vi "init.vi"(8 "error in":errorcluster, 10 "TBM module configuration in":refnum<class "TBM module configuration.lvclass">, 11 "dds runtime in":refnum<class "dds runtime.lvclass">) -> (0 "error out":errorcluster, 1 "data allocations":T1, 2 "execution settings":T4, 3 "dds runtime out":refnum<class "dds runtime.lvclass">)   [LabVIEW 2013, in "dds runtime.lvclass"]
doc: "Provides an interface for initializing a module at runtime. While this interface performs no operations, a child should provide an override which may open any necessary references or sessions, allocate necessary memory, and perform any final configuration validataion before providing the full configuration <b>execution data</b> to the calling process."
uses:
  dds runtime.lvclass
  <vilib>/NI/Tag Bus Module Framework/module configuration/TBM module configuration.lvclass
  <vilib>/NI/Tag Bus Module Framework/runtime/execution settings.ctl
  <vilib>/NI/Tag Bus Module Framework/channel/data tables.ctl
  <vilib>/NI/Tag Bus/dictionary/data dictionary.lvclass
  <vilib>/NI/Tag Bus/dictionary table pair.ctl
  <vilib>/NI/Tag Bus/table/data table.ctl
  configuration/dds configuration.lvclass
  configuration/dds configuration.lvclass/dds configuration.ctl
  <vilib>/NI/Tag Bus Module Framework/channel/TBM channel.lvclass/TBM channel.ctl
  dds runtime.lvclass/dds runtime.ctl
  <vilib>/NI/Tag Bus/tag/Data Type.ctl
  <vilib>/NI/Tag Bus/tag/tag descriptor.lvclass/tag descriptor.ctl
  <vilib>/RTI DDS Toolkit for LabVIEW/VIs/AdvancedCreateReader_NumDbl.vi
  <vilib>/RTI DDS Toolkit for LabVIEW/VIs/AdvancedCreateReader_NumSgl.vi
  <vilib>/RTI DDS Toolkit for LabVIEW/VIs/AdvancedCreateReader_NumI64.vi
  <vilib>/RTI DDS Toolkit for LabVIEW/VIs/AdvancedCreateReader_NumI32.vi
  <vilib>/RTI DDS Toolkit for LabVIEW/VIs/AdvancedCreateReader_NumI16.vi
  <vilib>/RTI DDS Toolkit for LabVIEW/VIs/AdvancedCreateReader_NumI8.vi
  <vilib>/RTI DDS Toolkit for LabVIEW/VIs/AdvancedCreateReader_NumU64.vi
  <vilib>/RTI DDS Toolkit for LabVIEW/VIs/AdvancedCreateReader_NumU32.vi
  <vilib>/RTI DDS Toolkit for LabVIEW/VIs/AdvancedCreateReader_NumU16.vi
  <vilib>/RTI DDS Toolkit for LabVIEW/VIs/AdvancedCreateReader_NumU8.vi
  <vilib>/RTI DDS Toolkit for LabVIEW/VIs/AdvancedCreateReader_Bool.vi
  <vilib>/RTI DDS Toolkit for LabVIEW/VIs/AdvancedCreateReader_String.vi
  <vilib>/RTI DDS Toolkit for LabVIEW/VIs/AdvancedCreateWriter_NumDbl.vi
  <vilib>/RTI DDS Toolkit for LabVIEW/VIs/AdvancedCreateWriter_NumSgl.vi
  <vilib>/RTI DDS Toolkit for LabVIEW/VIs/AdvancedCreateWriter_NumI64.vi
  <vilib>/RTI DDS Toolkit for LabVIEW/VIs/AdvancedCreateWriter_NumI32.vi
  <vilib>/RTI DDS Toolkit for LabVIEW/VIs/AdvancedCreateWriter_NumI16.vi
  <vilib>/RTI DDS Toolkit for LabVIEW/VIs/AdvancedCreateWriter_NumI8.vi
  <vilib>/RTI DDS Toolkit for LabVIEW/VIs/AdvancedCreateWriter_NumU64.vi
  <vilib>/RTI DDS Toolkit for LabVIEW/VIs/AdvancedCreateWriter_NumU32.vi
  <vilib>/RTI DDS Toolkit for LabVIEW/VIs/AdvancedCreateWriter_NumU16.vi
  <vilib>/RTI DDS Toolkit for LabVIEW/VIs/AdvancedCreateWriter_NumU8.vi
  <vilib>/RTI DDS Toolkit for LabVIEW/VIs/AdvancedCreateWriter_Bool.vi
  <vilib>/RTI DDS Toolkit for LabVIEW/VIs/AdvancedCreateWriter_String.vi
  <vilib>/NI/Tag Bus Module Framework/channel/TBM channel.lvclass
  <vilib>/NI/Tag Bus Module Framework/runtime/TBM module execution interface.lvclass
  <vilib>/NI/Tag Bus/tag/tag descriptor.lvclass
  <vilib>/RTI DDS Toolkit for LabVIEW/Library/LVDDS_library.lvlib
  <vilib>/NI/Tag Bus/tag bus.lvlib
  <vilib>/NI/Tag Bus/table/data table.lvlib
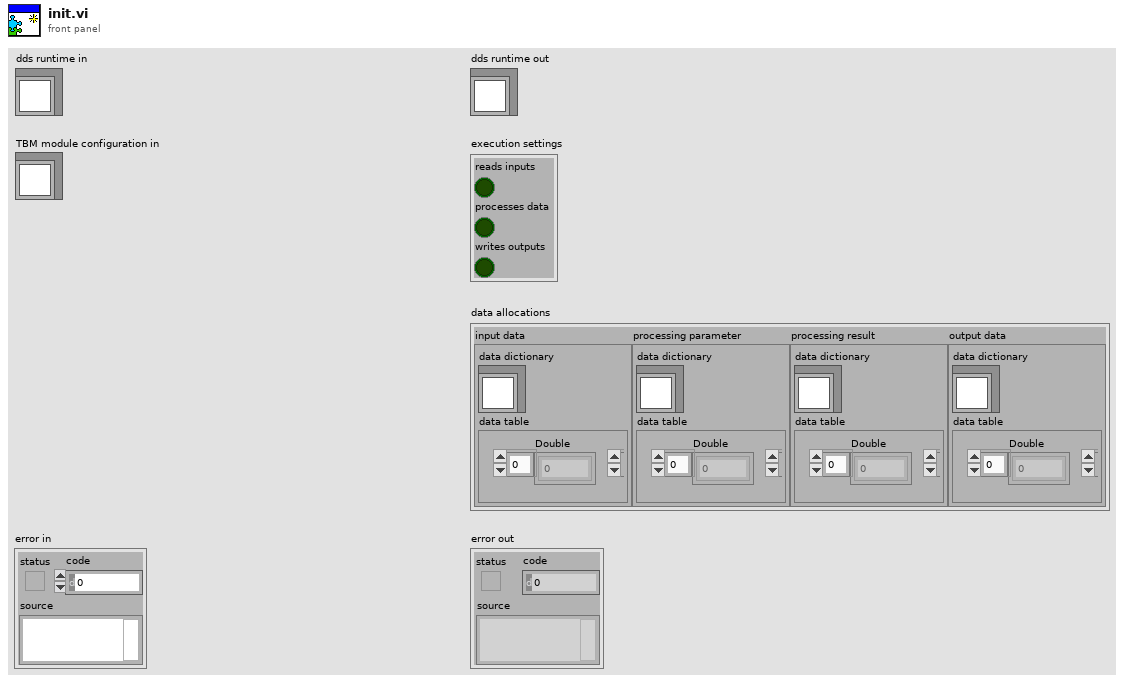
[diagram p1: front panel]
types:
  T1 = typedef "TBM channel.lvclass/data tables.ctl" = cluster{"input data":T2, "processing parameter":T2, "processing result":T2, "output data":T2}
  T2 = typedef "tag bus.lvlib/dictionary table pair.ctl" = cluster{"data dictionary":refnum<class "data dictionary.lvclass">, "data table":T3}
  T3 = typedef "tag bus.lvlib/data table.lvlib/data table.ctl" = cluster{"Double":dbl[], "Single":sgl[], "I64":i64[], "I32":i32[], "I16":i16[], "I8":i8[], "U64":u64[], "U32":u32[], "U16":u16[], "U8":u8[], "Boolean":bool[], "String":string[], "Array of Double":cluster{"DBL Array":dbl[]}[], "Array of Single":cluster{"SGL Array":sgl[]}[], "Array of I64":cluster{"I64 Array":i64[]}[], "Array of I32":cluster{"I32 Array":i32[]}[], "Array of I16":cluster{"I16 Array":i16[]}[], "Array of I8":cluster{"I8 Array":i8[]}[], "Array of U64":cluster{"U64 Array":u64[]}[], "Array of U32":cluster{"U32 Array":u32[]}[], "Array of U16":cluster{"U16 Array":u16[]}[], "Array of U8":cluster{"U8 Array":u8[]}[], "Array of Boolean":cluster{"Boolean Array":bool[]}[], "Array of String":cluster{"String Array":string[]}[]}
  T4 = typedef "TBM module execution interface.lvclass/execution settings.ctl" = cluster{"reads inputs":bool, "processes data":bool, "writes outputs":bool}
  T5 = typedef "tag bus.lvlib/tag descriptor.lvclass/Data Type.ctl" = enum16{"Double", "Single", "I64", "I32", "I16", "I8", "U64", "U32", "U16", "U8", "Boolean", "String", "Array of Double", "Array of Single", "Array of I64", "Array of I32", "Array of I16", "Array of I8", "Array of U64", "Array of U32", "Array of U16", "Array of U8", "Array of Boolean", "Array of String"}
  T6 = cluster{"index":i32, "data type":T5, "ref num":u64, "new samples only":bool, "query condition":string}
  T7 = cluster{"index":i32, "data type":T5, "ref num":u64}
  T8 = typedef "dds configuration.lvclass/Line.ctl" = cluster{"channel":refnum<class "TBM channel.lvclass">, "DDS topic":string, "DDS Domain":u32, "advanced configuration":T9}
  T9 = typedef "LVDDS_library.lvlib/RTI DDS Advanced Reader Configuration.ctl" = cluster{"typeName":string, "keyName":string, "domainParticipantQoSProfile":string, "dataReaderQoSProfile":string, "forceNewDomainParticipant?":bool, "forceArrayMapping?":bool, "forceExclusiveReader?":bool, "forceRead? (only ExclusiveReader)":bool, "forceUnboundedString?":bool}
  T10 = typedef "TBM channel.lvclass/channel classification.ctl" = enum16{"input data", "output data", "processing parameter", "processing result"}
  T11 = cluster{"index":i32, "data type":T5, "ref num":u64, "new samples only":bool, "query condition":string}[]
  T12 = cluster{"index":i32, "data type":T5, "ref num":u64}[]
  T13 = typedef "LVDDS_library.lvlib/RTI DDS Advanced Writer Configuration.ctl" = cluster{"typeName":string, "keyName":string, "domainParticipantQoSProfile":string, "dataWriterQoSProfile":string, "forceNewDomainParticipant?":bool, "forceArrayMapping?":bool, "forceUnboundedString?":bool}
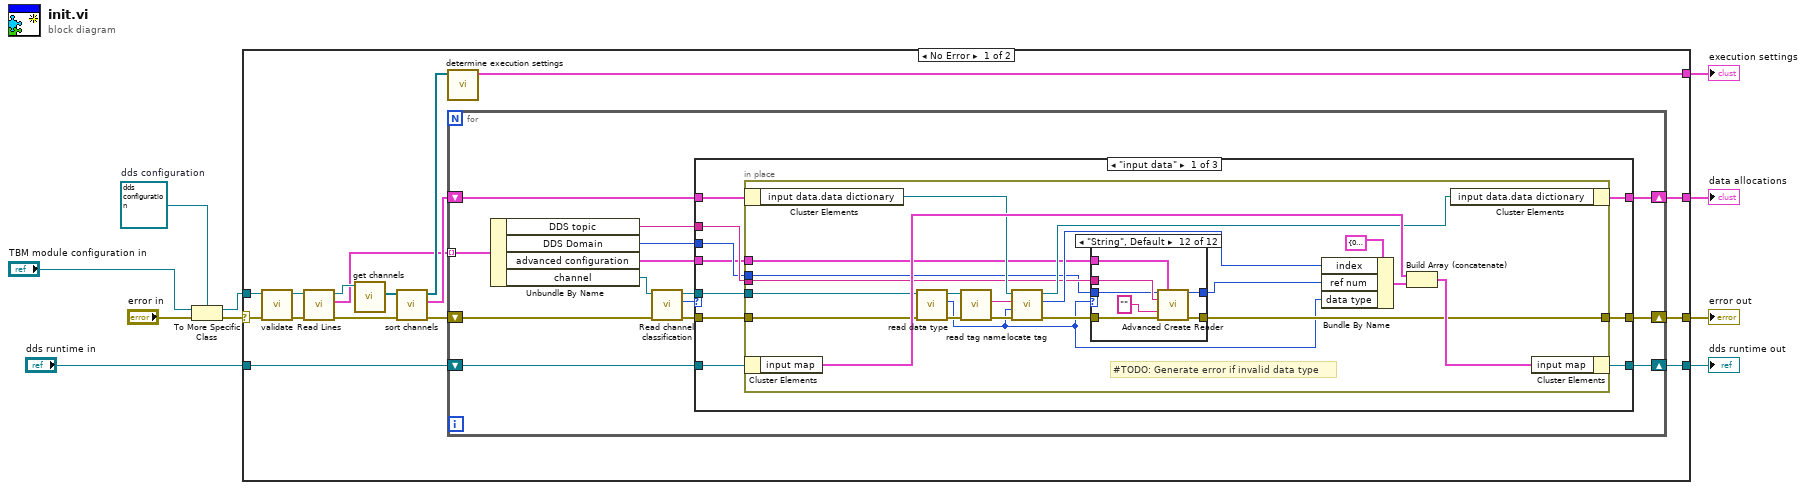
[diagram p0: block diagram]
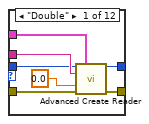
[diagram p2: hidden frame]
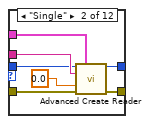
[diagram p3: hidden frame]
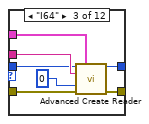
[diagram p4: hidden frame]
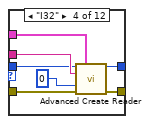
[diagram p5: hidden frame]
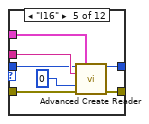
[diagram p6: hidden frame]
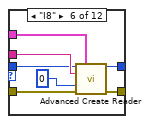
[diagram p7: hidden frame]
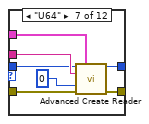
[diagram p8: hidden frame]
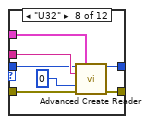
[diagram p9: hidden frame]
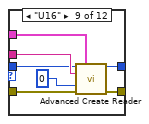
[diagram p10: hidden frame]
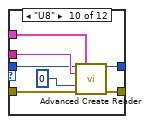
[diagram p11: hidden frame]
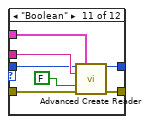
[diagram p12: hidden frame]
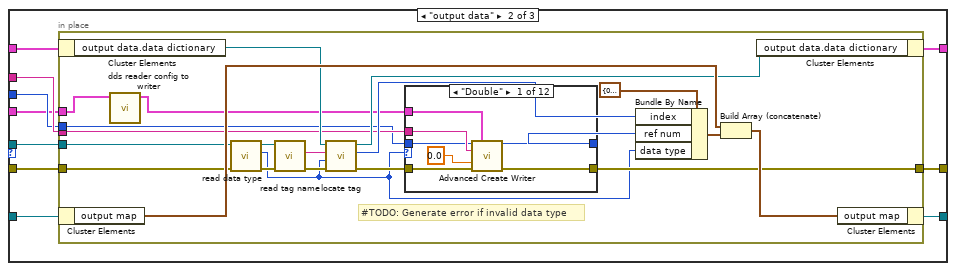
[diagram p13: hidden frame]
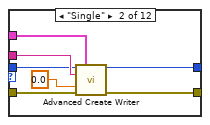
[diagram p14: hidden frame]
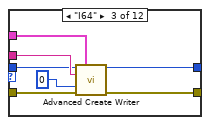
[diagram p15: hidden frame]
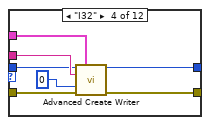
[diagram p16: hidden frame]
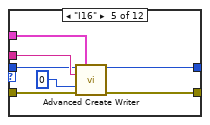
[diagram p17: hidden frame]
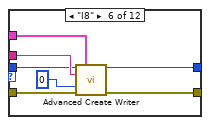
[diagram p18: hidden frame]
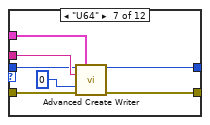
[diagram p19: hidden frame]
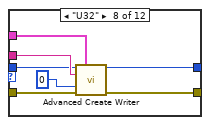
[diagram p20: hidden frame]
diagram:
  w8 = refnum<class "dds configuration.lvclass"> refnum  # dds configuration
  n1 = To More Specific Class(target class=w8, reference="TBM module configuration in", error in="error in") -> (specific class reference=w9:refnum<class "dds configuration.lvclass">, error out=w10:errorcluster)
  n2 = case shown="No Error" w10 {
    selector: w10 -> [w25 w273]
    tunnel: w9 -> [w24 _]
    tunnel: "dds runtime in" -> [w23 w274]
    tunnel: [w22 w274] -> w4
    tunnel: [w12 w273] -> w3
    tunnel: [w11 _] -> w1
    tunnel: [w26 _] -> w2
    frame No Error {
      n3 = call-dynamic "validate.vi"("error in"=w25, "dds configuration in"=w24) -> ("error out"=w17:errorcluster, "dds configuration out"=w18:refnum<class "dds configuration.lvclass">)  [unwired: 8 in]
      n4 = call "Read Lines.vi"("error in (no error)"=w17, "dds configuration in"=w18) -> ("error out"=w16:errorcluster, "Lines"=w14:T8[], "dds configuration out"=w15:refnum<class "dds configuration.lvclass">)  [unwired: 7 in]
      n5 = call-dynamic "get channels.vi"("dds configuration in"=w15) -> ("channels"=w21:refnum<class "TBM channel.lvclass">[])  [unwired: 9 in, 1 out]
      n6 = call <vilib>:"sort channels.vi"("error in"=w16, "channels in"=w21) -> ("error out"=w13:errorcluster, "data allocations"=w19:T1, "channels out"=w20:refnum<class "TBM channel.lvclass">[])  [unwired: 7 in]
      n7 = call <vilib>:"determine execution settings.vi"("channels"=w20) -> ("execution settings"=w26:T4)  [unwired: 10 in]
      n8 = for {
        shift-right: [w37] -> w22
        shift-left: w23 -> [w40]
        tunnel: w14 -> [w34] mode=indexing
        shift-right: [w29] -> w12
        shift-left: w13 -> [w30]
        shift-right: [w27] -> w11
        shift-left: w19 -> [w35]
        n9 = Unbundle By Name(w34) -> ("DDS topic"=w33:string, "DDS Domain"=w32:u32, "advanced configuration"=w31:T9, "channel"=w28:refnum<class "TBM channel.lvclass">)
        n10 = call <vilib>:"Read channel classification.vi"("error in"=w30, "channel in"=w28) -> ("error out"=w36:errorcluster, "channel classification"=w39:T10, "channel out"=w38:refnum<class "TBM channel.lvclass">)  [unwired: 7 in]
        n11 = case shown="\"input data\"" w39 {
          tunnel: w40 -> [w50 w164 w270]
          tunnel: w38 -> [w47 w161 _]
          tunnel: [w49 w163 w270] -> w37
          tunnel: w36 -> [w48 w162 w271]
          tunnel: w35 -> [w46 w160 w272]
          tunnel: w33 -> [w45 w159 _]
          tunnel: w32 -> [w44 w158 _]
          tunnel: w31 -> [w43 w157 _]
          tunnel: [w42 w156 w271] -> w29
          tunnel: [w41 w155 w272] -> w27
          frame "input data" {
            n12 = in-place {
              in-place-border: w48 -> [w68]
              in-place-border: w47 -> [w66]
              in-place-border: w45 -> [w58]
              in-place-border: w44 -> [w57]
              in-place-border: w43 -> [w56]
              in-place-border: [w54] -> w42
              # "#TODO: Generate error if invalid data type"
              n13 = in-place-cluster #1(w46) -> ("input data.data dictionary"=w65:refnum<class "data dictionary.lvclass">)
              n14 = in-place-cluster #2(w50) -> ("input map"=w70:T11)
              n15 = call <vilib>:"read data type.vi"("error in"=w68, "system tag in"=w66) -> ("error out"=w62:errorcluster, "data type"=w52:T5, "system tag out"=w63:refnum<class "TBM channel.lvclass">)  [unwired: 7 in]
              n16 = call <vilib>:"read tag name.vi"("error in"=w62, "system tag in"=w63) -> ("error out"=w55:errorcluster, "name"=w61:string)  [unwired: 7 in, 1 out]
              n17 = call <vilib>:"locate tag.vi"("error in"=w55, "data type"=w52, "name"=w61, "data dictionary in"=w65) -> ("error out"=w60:errorcluster, "index"=w59:i32, "data dictionary out"=w64:refnum<class "data dictionary.lvclass">)  [unwired: 5 in]
              n18 = case shown="\"String\", Default" w52 {
                tunnel: [w77 w84 w91 w98 w105 w112 w119 w126 w133 w140 w147 w154] -> w53
                tunnel: w60 -> [w75 w82 w89 w96 w103 w110 w117 w124 w131 w138 w145 w152]
                tunnel: [w74 w81 w88 w95 w102 w109 w116 w123 w130 w137 w144 w151] -> w54
                tunnel: w58 -> [w73 w80 w87 w94 w101 w108 w115 w122 w129 w136 w143 w150]
                tunnel: w57 -> [w72 w79 w86 w93 w100 w107 w114 w121 w128 w135 w142 w149]
                tunnel: w56 -> [w71 w78 w85 w92 w99 w106 w113 w120 w127 w134 w141 w148]
                frame "Double" {
                  n19 = call-poly <vilib>:"Advanced Create Reader.vi"("domain id"=w72, "advanced reader configuration"=w71, "topic name"=w73, "data type"=0.0, "error in (no error)"=w75) -> ("ref num"=w77:u64, "error out"=w74:errorcluster)  [unwired: 9 in]
                }
                frame "Single" {
                  n20 = call-poly <vilib>:"Advanced Create Reader.vi"("domain id"=w79, "advanced reader configuration"=w78, "topic name"=w80, "data type"=sgl 0.0, "error in (no error)"=w82) -> ("ref num"=w84:u64, "error out"=w81:errorcluster)  [unwired: 9 in]
                }
                frame "I64" {
                  n21 = call-poly <vilib>:"Advanced Create Reader.vi"("domain id"=w86, "advanced reader configuration"=w85, "topic name"=w87, "data type"=i64 0, "error in (no error)"=w89) -> ("ref num"=w91:u64, "error out"=w88:errorcluster)  [unwired: 9 in]
                }
                frame "I32" {
                  n22 = call-poly <vilib>:"Advanced Create Reader.vi"("domain id"=w93, "advanced reader configuration"=w92, "topic name"=w94, "data type"=0, "error in (no error)"=w96) -> ("ref num"=w98:u64, "error out"=w95:errorcluster)  [unwired: 9 in]
                }
                frame "I16" {
                  n23 = call-poly <vilib>:"Advanced Create Reader.vi"("domain id"=w100, "advanced reader configuration"=w99, "topic name"=w101, "data type"=i16 0, "error in (no error)"=w103) -> ("ref num"=w105:u64, "error out"=w102:errorcluster)  [unwired: 9 in]
                }
                frame "I8" {
                  n24 = call-poly <vilib>:"Advanced Create Reader.vi"("domain id"=w107, "advanced reader configuration"=w106, "topic name"=w108, "data type"=i8 0, "error in (no error)"=w110) -> ("ref num"=w112:u64, "error out"=w109:errorcluster)  [unwired: 9 in]
                }
                frame "U64" {
                  n25 = call-poly <vilib>:"Advanced Create Reader.vi"("domain id"=w114, "advanced reader configuration"=w113, "topic name"=w115, "data type"=u64 0, "error in (no error)"=w117) -> ("ref num"=w119:u64, "error out"=w116:errorcluster)  [unwired: 9 in]
                }
                frame "U32" {
                  n26 = call-poly <vilib>:"Advanced Create Reader.vi"("domain id"=w121, "advanced reader configuration"=w120, "topic name"=w122, "data type"=u32 0, "error in (no error)"=w124) -> ("ref num"=w126:u64, "error out"=w123:errorcluster)  [unwired: 9 in]
                }
                frame "U16" {
                  n27 = call-poly <vilib>:"Advanced Create Reader.vi"("domain id"=w128, "advanced reader configuration"=w127, "topic name"=w129, "data type"=u16 0, "error in (no error)"=w131) -> ("ref num"=w133:u64, "error out"=w130:errorcluster)  [unwired: 9 in]
                }
                frame "U8" {
                  n28 = call-poly <vilib>:"Advanced Create Reader.vi"("domain id"=w135, "advanced reader configuration"=w134, "topic name"=w136, "data type"=u8 0, "error in (no error)"=w138) -> ("ref num"=w140:u64, "error out"=w137:errorcluster)  [unwired: 9 in]
                }
                frame "Boolean" {
                  n29 = call-poly <vilib>:"Advanced Create Reader.vi"("domain id"=w142, "advanced reader configuration"=w141, "topic name"=w143, "data type"=FALSE, "error in (no error)"=w145) -> ("ref num"=w147:u64, "error out"=w144:errorcluster)  [unwired: 9 in]
                }
                frame "String", Default {
                  n30 = call-poly <vilib>:"Advanced Create Reader.vi"("domain id"=w149, "advanced reader configuration"=w148, "topic name"=w150, "data type"="", "error in (no error)"=w152) -> ("ref num"=w154:u64, "error out"=w151:errorcluster)  [unwired: 9 in]
                }
              }
              n31 = Bundle By Name(cluster=T6 {"index"=0, "data type"=enum."Double", "ref num"=0, "new samples only"=FALSE, "query condition"=""} ("item"), "index"=w59, "ref num"=w53, "data type"=w52) -> (w67:T6)
              n32 = Build Array (concatenate)(w70, w67) -> (w69:T11)
              n33 = in-place-cluster #1("input data.data dictionary"=w64) -> (w41:T1)
              n34 = in-place-cluster #2("input map"=w69) -> (w49:refnum<class "dds runtime.lvclass">)
            }
          }
          frame "output data" {
            n35 = in-place {
              in-place-border: w162 -> [w183]
              in-place-border: w161 -> [w180]
              in-place-border: w159 -> [w172]
              in-place-border: w158 -> [w171]
              in-place-border: w157 -> [w166]
              in-place-border: [w169] -> w156
              # "#TODO: Generate error if invalid data type"
              n36 = in-place-cluster #3(w160) -> ("output data.data dictionary"=w179:refnum<class "data dictionary.lvclass">)
              n37 = in-place-cluster #4(w164) -> ("output map"=w185:T12)
              n38 = call "dds reader config to writer.vi"("reader configuration"=w166) -> ("writer configuration"=w165:T13)  [unwired: 10 in]
              n39 = call <vilib>:"read data type.vi"("error in"=w183, "system tag in"=w180) -> ("error out"=w176:errorcluster, "data type"=w167:T5, "system tag out"=w177:refnum<class "TBM channel.lvclass">)  [unwired: 7 in]
              n40 = call <vilib>:"read tag name.vi"("error in"=w176, "system tag in"=w177) -> ("error out"=w170:errorcluster, "name"=w175:string)  [unwired: 7 in, 1 out]
              n41 = call <vilib>:"locate tag.vi"("error in"=w170, "data type"=w167, "name"=w175, "data dictionary in"=w179) -> ("error out"=w174:errorcluster, "index"=w173:i32, "data dictionary out"=w178:refnum<class "data dictionary.lvclass">)  [unwired: 5 in]
              n42 = case shown="\"Double\"" w167 {
                tunnel: [w192 w199 w206 w213 w220 w227 w234 w241 w248 w255 w262 w269] -> w168
                tunnel: w174 -> [w190 w197 w204 w211 w218 w225 w232 w239 w246 w253 w260 w267]
                tunnel: [w189 w196 w203 w210 w217 w224 w231 w238 w245 w252 w259 w266] -> w169
                tunnel: w172 -> [w188 w195 w202 w209 w216 w223 w230 w237 w244 w251 w258 w265]
                tunnel: w171 -> [w187 w194 w201 w208 w215 w222 w229 w236 w243 w250 w257 w264]
                tunnel: w165 -> [w186 w193 w200 w207 w214 w221 w228 w235 w242 w249 w256 w263]
                frame "Double" {
                  n43 = call-poly <vilib>:"Advanced Create Writer.vi"("domain id"=w187, "advanced writer configuration"=w186, "topic name"=w188, "data type"=0.0, "error in (no error)"=w190) -> ("ref num"=w192:u64, "error out"=w189:errorcluster)  [unwired: 9 in]
                }
                frame "Single" {
                  n44 = call-poly <vilib>:"Advanced Create Writer.vi"("domain id"=w194, "advanced writer configuration"=w193, "topic name"=w195, "data type"=sgl 0.0, "error in (no error)"=w197) -> ("ref num"=w199:u64, "error out"=w196:errorcluster)  [unwired: 9 in]
                }
                frame "I64" {
                  n45 = call-poly <vilib>:"Advanced Create Writer.vi"("domain id"=w201, "advanced writer configuration"=w200, "topic name"=w202, "data type"=i64 0, "error in (no error)"=w204) -> ("ref num"=w206:u64, "error out"=w203:errorcluster)  [unwired: 9 in]
                }
                frame "I32" {
                  n46 = call-poly <vilib>:"Advanced Create Writer.vi"("domain id"=w208, "advanced writer configuration"=w207, "topic name"=w209, "data type"=0, "error in (no error)"=w211) -> ("ref num"=w213:u64, "error out"=w210:errorcluster)  [unwired: 9 in]
                }
                frame "I16" {
                  n47 = call-poly <vilib>:"Advanced Create Writer.vi"("domain id"=w215, "advanced writer configuration"=w214, "topic name"=w216, "data type"=i16 0, "error in (no error)"=w218) -> ("ref num"=w220:u64, "error out"=w217:errorcluster)  [unwired: 9 in]
                }
                frame "I8" {
                  n48 = call-poly <vilib>:"Advanced Create Writer.vi"("domain id"=w222, "advanced writer configuration"=w221, "topic name"=w223, "data type"=i8 0, "error in (no error)"=w225) -> ("ref num"=w227:u64, "error out"=w224:errorcluster)  [unwired: 9 in]
                }
                frame "U64" {
                  n49 = call-poly <vilib>:"Advanced Create Writer.vi"("domain id"=w229, "advanced writer configuration"=w228, "topic name"=w230, "data type"=u64 0, "error in (no error)"=w232) -> ("ref num"=w234:u64, "error out"=w231:errorcluster)  [unwired: 9 in]
                }
                frame "U32" {
                  n50 = call-poly <vilib>:"Advanced Create Writer.vi"("domain id"=w236, "advanced writer configuration"=w235, "topic name"=w237, "data type"=u32 0, "error in (no error)"=w239) -> ("ref num"=w241:u64, "error out"=w238:errorcluster)  [unwired: 9 in]
                }
                frame "U16" {
                  n51 = call-poly <vilib>:"Advanced Create Writer.vi"("domain id"=w243, "advanced writer configuration"=w242, "topic name"=w244, "data type"=u16 0, "error in (no error)"=w246) -> ("ref num"=w248:u64, "error out"=w245:errorcluster)  [unwired: 9 in]
                }
                frame "U8" {
                  n52 = call-poly <vilib>:"Advanced Create Writer.vi"("domain id"=w250, "advanced writer configuration"=w249, "topic name"=w251, "data type"=u8 0, "error in (no error)"=w253) -> ("ref num"=w255:u64, "error out"=w252:errorcluster)  [unwired: 9 in]
                }
                frame "Boolean" {
                  n53 = call-poly <vilib>:"Advanced Create Writer.vi"("domain id"=w257, "advanced writer configuration"=w256, "topic name"=w258, "data type"=FALSE, "error in (no error)"=w260) -> ("ref num"=w262:u64, "error out"=w259:errorcluster)  [unwired: 9 in]
                }
                frame "String", Default {
                  n54 = call-poly <vilib>:"Advanced Create Writer.vi"("domain id"=w264, "advanced writer configuration"=w263, "topic name"=w265, "data type"="", "error in (no error)"=w267) -> ("ref num"=w269:u64, "error out"=w266:errorcluster)  [unwired: 9 in]
                }
              }
              n55 = Bundle By Name(cluster=T7 {"index"=0, "data type"=enum."Double", "ref num"=0} ("item"), "index"=w173, "ref num"=w168, "data type"=w167) -> (w181:T7)
              n56 = Build Array (concatenate)(w185, w181) -> (w184:T12)
              n57 = in-place-cluster #3("output data.data dictionary"=w178) -> (w155:T1)
              n58 = in-place-cluster #4("output map"=w184) -> (w163:refnum<class "dds runtime.lvclass">)
            }
          }
          frame Default {
          }
        }
      }
    }
    frame Error {
    }
  }
  "error out" <- w3
  "dds runtime out" <- w4
  "execution settings" <- w2
  "data allocations" <- w1
